vi "Birch.vi"(8 "error in":errorcluster) -> (0 "error out":errorcluster, 3 "out":refnum<class "Birch.lvclass">)   [LabVIEW 2020]
doc: "Implements the BIRCH clustering algorithm.\n\n It is a memory-efficient, online-learning algorithm provided as an\n alternative to :class:`MiniBatchKMeans`. It constructs a tree\n data structure with the cluster centroids being read off the leaf.\n These can be either the final cluster centroids or can be provided as input\n to another clustering algorithm such as :class:`AgglomerativeClustering`.\n\n Read more in the :ref:`User Guide <birch>`.\n\n .. versionadded:: 0.16\n\n Parameters\n ----------\n threshold : float, default=0.5\n The radius of the subcluster obtained by merging a new sample and the\n closest subcluster should be lesser than the threshold. Otherwise a new\n subcluster is started. Setting this value to be very low promotes\n splitting and vice-versa.\n\n branching_factor : int, default=50\n Maximum number of CF subclusters in each node. If a new samples enters\n such that the number of subclusters exceed the branching_factor then\n that node is split into two nodes with the subclusters redistributed\n in each. The parent subcluster of that node is removed and two new\n subclusters are added as parents of the 2 split nodes.\n\n n_clusters : int, instance of sklearn.cluster model, default=3\n Number of clusters after the final clustering step, which treats the\n subclusters from the leaves as new samples.\n\n - `None` : the final clustering step is not performed and the\n subclusters are returned as they are.\n\n - :mod:`sklearn.cluster` Estimator : If a model is provided, the model\n is fit treating the subclusters as new samples and the initial data\n is mapped to the label of the closest subcluster.\n\n - `int` : the model fit is :class:`AgglomerativeClustering` with\n `n_clusters` set to be equal to the int.\n\n compute_labels : bool, default=True\n Whether or not to compute labels for each fit.\n\n copy : bool, default=True\n Whether or not to make a copy of the given data. If set to False,\n the initial data will be overwritten.\n\n Attributes\n ----------\n root_ : _CFNode\n Root of the CFTree.\n\n dummy_leaf_ : _CFNode\n Start pointer to all the leaves.\n\n subcluster_centers_ : ndarray\n Centroids of all subclusters read directly from the leaves.\n\n subcluster_labels_ : ndarray\n Labels assigned to the centroids of the subclusters after\n they are clustered globally.\n\n labels_ : ndarray of shape (n_samples,)\n Array of labels assigned to the input data.\n if partial_fit is used instead of fit, they are assigned to the\n last batch of data.\n\n See Also\n --------\n MiniBatchKMeans : Alternative implementation that does incremental updates\n of the centers' positions using mini-batches.\n\n Notes\n -----\n The tree data structure consists of nodes with each node consisting of\n a number of subclusters. The maximum number of subclusters in a node\n is determined by the branching factor. Each subcluster maintains a\n linear sum, squared sum and the number of samples in that subcluster.\n In addition, each subcluster can also have a node as its child, if the\n subcluster is not a member of a leaf node.\n\n For a new point entering the root, it is merged with the subcluster closest\n to it and the linear sum, squared sum and the number of samples of that\n subcluster are updated. This is done recursively till the properties of\n the leaf node are updated.\n\n References\n ----------\n * Tian Zhang, Raghu Ramakrishnan, Maron Livny\n BIRCH: An efficient data clustering method for large databases.\n https://www.cs.sfu.ca/CourseCentral/459/han/papers/zhang96.pdf\n\n * Roberto Perdisci\n JBirch - Java implementation of BIRCH clustering algorithm\n https://code.google.com/archive/p/jbirch\n\n \nAvailable methods:\nGet Attributes\nGet Params\nSet Params"
uses:
  Birch.lvclass
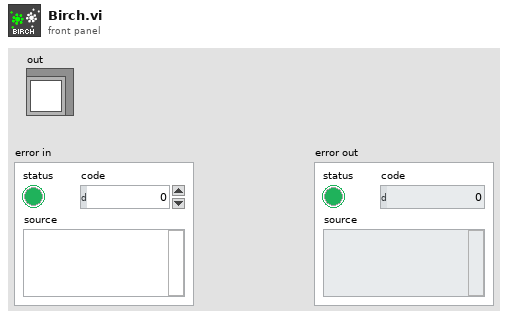
[diagram p1: front panel]
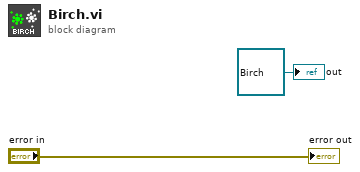
[diagram p0: block diagram]
diagram:
  "out" <- refnum<class "Birch.lvclass"> refnum ("model")
  "error out" <- "error in"
